vi "FlowHzToGPM.vi"(8 "error in":errorcluster, 9 "GPM":dbl[](array[numeric])=[0.0, 0.01403, 0.0282, 0.04999, 0.10258, 0.2127, 0.29025, 0.38705, 0.4802, 0.58116, 0.67343, 0.78891, 0.88241, 0.99458, 1.0892, 1.18752, 1.40024, 1.49696, 1.61641, 1.82395, 2.03827], 10 "Hz":dbl[](array[numeric])=[0.0, 3.61, 7.37, 13.09, 27.01, 55.78, 75.99, 100.94, 124.81, 150.52, 173.77, 202.7, 225.93, 253.45, 276.83, 301.27, 352.82, 375.82, 403.94, 453.6, 503.78], 11 "Freq":dbl) -> (0 "error out":errorcluster, 2 "Flow Hz":dbl, 3 "FlowGPH":dbl)   [LabVIEW 2018]
uses:
  <vilib>/Analysis/baseanly.llb/Mean (DBL).vi
  <vilib>/measure/macond.llb/FIR Filter for 1 Chan.vi
  <vilib>/gmath/NI_Gmath.lvlib
  <vilib>/measure/NI_MAPro.lvlib
  <vilib>/Analysis/NI_AALBase.lvlib
panel:
  out "Buffer Full":bool
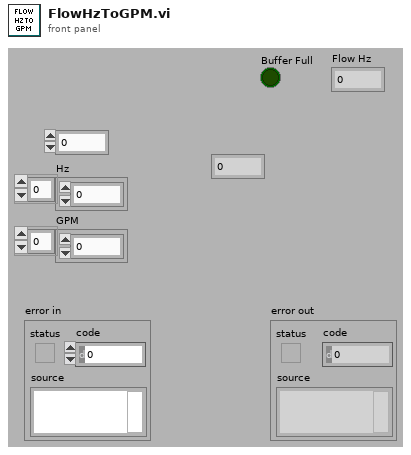
[diagram p1: front panel]
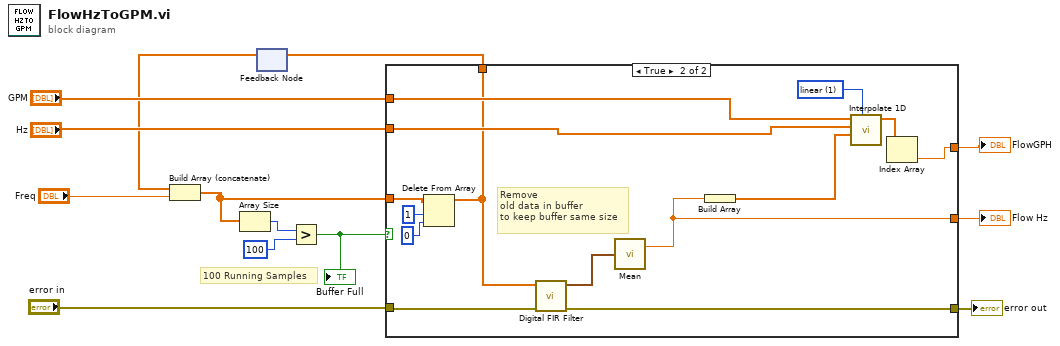
[diagram p0: block diagram]
diagram:
  # "100 Running Samples"
  n1 = feedback #1() -> (w7:dbl[])  [unwired: 1 in]
  n2 = Build Array (concatenate)(w7, "Freq") -> (w4:dbl[])
  n3 = Array Size(array=w4) -> (size(s)=w6:i32)
  n4 = Greater?(x=w6, y=100) -> (0:w2:bool)
  "Buffer Full" <- w2
  n5 = case shown="True" w2 {
    tunnel: [_ w29] -> w13
    tunnel: [_ w28] -> w12
    tunnel: "GPM" -> [_ w27]
    tunnel: "Hz" -> [_ w26]
    tunnel: w4 -> [w15 w21]
    tunnel: [w15 w16] -> w3
    tunnel: "error in" -> [w14 w18]
    tunnel: [w14 w17] -> w8
    frame False {
    }
    frame True {
      w25 = 1 items=["nearest", "linear", "spline", "cubic Hermite", "Lagrange"] ("method")
      # "Remove\nold data in buffer\nto keep buffer same size"
      n6 = Delete From Array(array=w21, length=1, index=0) -> (array with subset deleted=w16:dbl[])  [unwired: 1 out]
      n7 = call-poly <vilib>:"Digital FIR Filter.vi"("error in (no error)"=w18, "signal in"=w16) -> ("error out"=w17:errorcluster, "signal out"=w22:waveform(dbl))  [unwired: 7 in, 1 out]
      n8 = call-poly <vilib>:"Mean.vi"("X"=w22) -> ("mean"=w28:dbl)  [unwired: 1 out]
      n9 = Build Array(w28) -> (w23:dbl[])
      n10 = call <vilib>:"Interpolate 1D.vi"("method"=w25, "xi"=w23, "X"=w26, "Y"=w27) -> ("yi"=w24:dbl[])  [unwired: 5 in, 2 out]
      n11 = Index Array(array=w24) -> (element=w29:dbl)  [unwired: 1 in]
    }
  }
  "error out" <- w8
  "FlowGPH" <- w13
  "Flow Hz" <- w12
  n12 = feedback-in #1(w3) -> ()
